vi "WordToHex.vi"(11 "WORD":u16[](array[numeric])) -> (3 "数组":u16[](array[numeric]) format="%04xH")   [LabVIEW 2016, in "挥发酚.lvlib"]
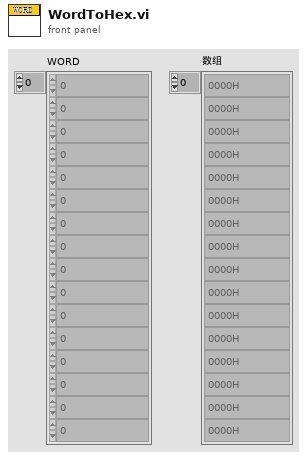
[diagram p1: front panel]
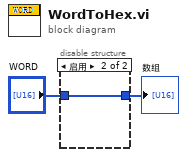
[diagram p0: block diagram]
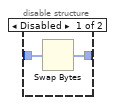
[diagram p2: hidden frame]
diagram:
  n1 = disable-structure shown="启用" {
    disable-tunnel: "WORD" -> [w4 w5]
    disable-tunnel: [w3 w5] -> w1
    frame Disabled {
      n2 = Swap Bytes(anything=w4) -> (byte swapped=w3:u16[])
    }
    frame Enabled {
    }
  }
  "数组" <- w1
